vi "Get Low Terminals Connection.vi"(8 "error in (no error)":errorcluster, 11 "VISA resource name":refnum<visa-resource-name>) -> (0 "error out":errorcluster, 2 "Low Terminals Connection":u16, 3 "VISA resource name out":refnum<visa-resource-name>)   [LabVIEW 2014, in "Fluke 5XXX Series Multicalibrators.lvlib"]
doc: "This VI returns whether or not the Calibrator front panel NORMAL LO terminal and AUX LO terminal are internally tied together (default) or are open.\n\nNote:\n\nThis VI is available only for instrument models 5500A and 5520A."
uses:
  Fluke 5XXX Series Multicalibrators.lvlib
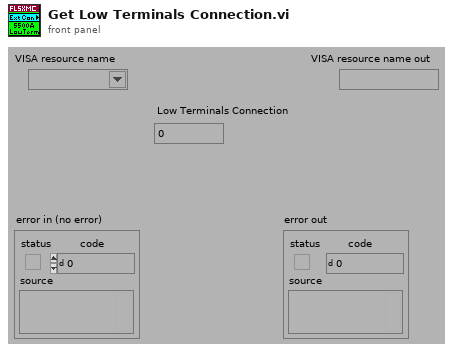
[diagram p1: front panel]
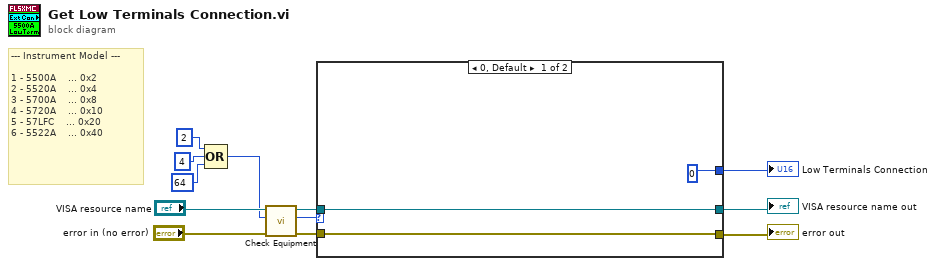
[diagram p0: block diagram]
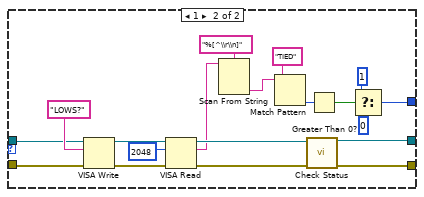
[diagram p2: hidden frame]
diagram:
  # "--- Instrument Model ---\n\n1 - 5500A    ... 0x2\n2 - 5520A    ... 0x4\n3 - 5700A    ... 0x8\n4 - 5720A    ... 0x10\n5 - 57LFC    ... 0x20\n6 - 5522A    ... 0x40"
  n1 = Compound Arithmetic op=OR(2 ("Numeric"), 4 ("Numeric"), 64 ("Numeric")) -> (w4:i32)
  n2 = call "Check Equipment.vi"("error in (no error)"="error in (no error)", "Bit Mask"=w4, "VISA resource name"="VISA resource name") -> ("error out"=w12:errorcluster, "Present?"=w11:u32, "VISA resource name out"=w10:refnum<visa-resource-name>)  [unwired: 6 in]
  n3 = case shown="0, Default" w11 {
    tunnel: [w14 w28] -> w9
    tunnel: [w13 w25] -> w8
    tunnel: w12 -> [w14 w30]
    tunnel: w10 -> [w13 w29]
    tunnel: [u16 0 w16] -> w7
    frame 0, Default {
    }
    frame 1 {
      n4 = VISA Write(VISA resource name=w29, write buffer="LOWS?", error in (no error)=w30) -> (VISA resource name out=w33:refnum<visa-resource-name>, error out=w32:errorcluster)  [unwired: 1 out]
      n5 = VISA Read(VISA resource name=w33, byte count=u32 2048 ("byte count (0)"), error in (no error)=w32) -> (VISA resource name out=w26:refnum<visa-resource-name>, read buffer=w18:string, error out=w27:errorcluster)  [unwired: 1 out]
      n6 = Scan From String(format string="%[^\\r\\n]", input string=w18) -> (output 1=w17:string)  [unwired: 3 in, 3 out]
      n7 = Match Pattern(string=w17, regular expression="TIED") -> (offset past match=w22:i32)  [unwired: 1 in, 3 out]
      n8 = call "Check Status.vi"("VISA resource name"=w26, "error in (no error)"=w27) -> ("VISA resource name out"=w25:refnum<visa-resource-name>, "error out"=w28:errorcluster)  [unwired: 12 in]
      n9 = Greater Than 0?(x=w22) -> (x > 0?=w19:bool)
      n10 = Select(t=u16 1 ("f"), s=w19, f=u16 0) -> (s? t:f=w16:u16)
    }
  }
  "Low Terminals Connection" <- w7
  "VISA resource name out" <- w8
  "error out" <- w9
